vi "LAB3.vi"() -> ()   [LabVIEW 2015]
panel:
  in  "CH2":bool
  in  "CH1":bool
  in  "Enable CH":bool
  out "chaîne résultante 3":string
  out "chaîne résultante 2":string
  out "chaîne en sortie":string
  out "chaîne résultante":string
  out "sortie d'erreur":errorcluster
  in  "Frequency":dbl
  in  "Unit":u16(ring) items=["VPP", "VRMS", "DBM"]
  in  "DC Offset":dbl
  in  "Stop":bool
  in  "Amplitude":dbl
  in  "Waveform":u16(ring) items=["DC", "Sine", "Square", "Ramp", "Pulse", "Noise", "Arb"]
  in  "Configurer":bool
  in  "Nom de ressource VISA":refnum<visa-resource-name>
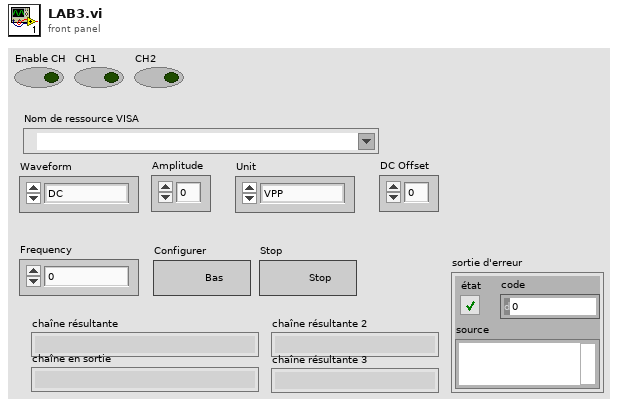
[diagram p1: front panel]
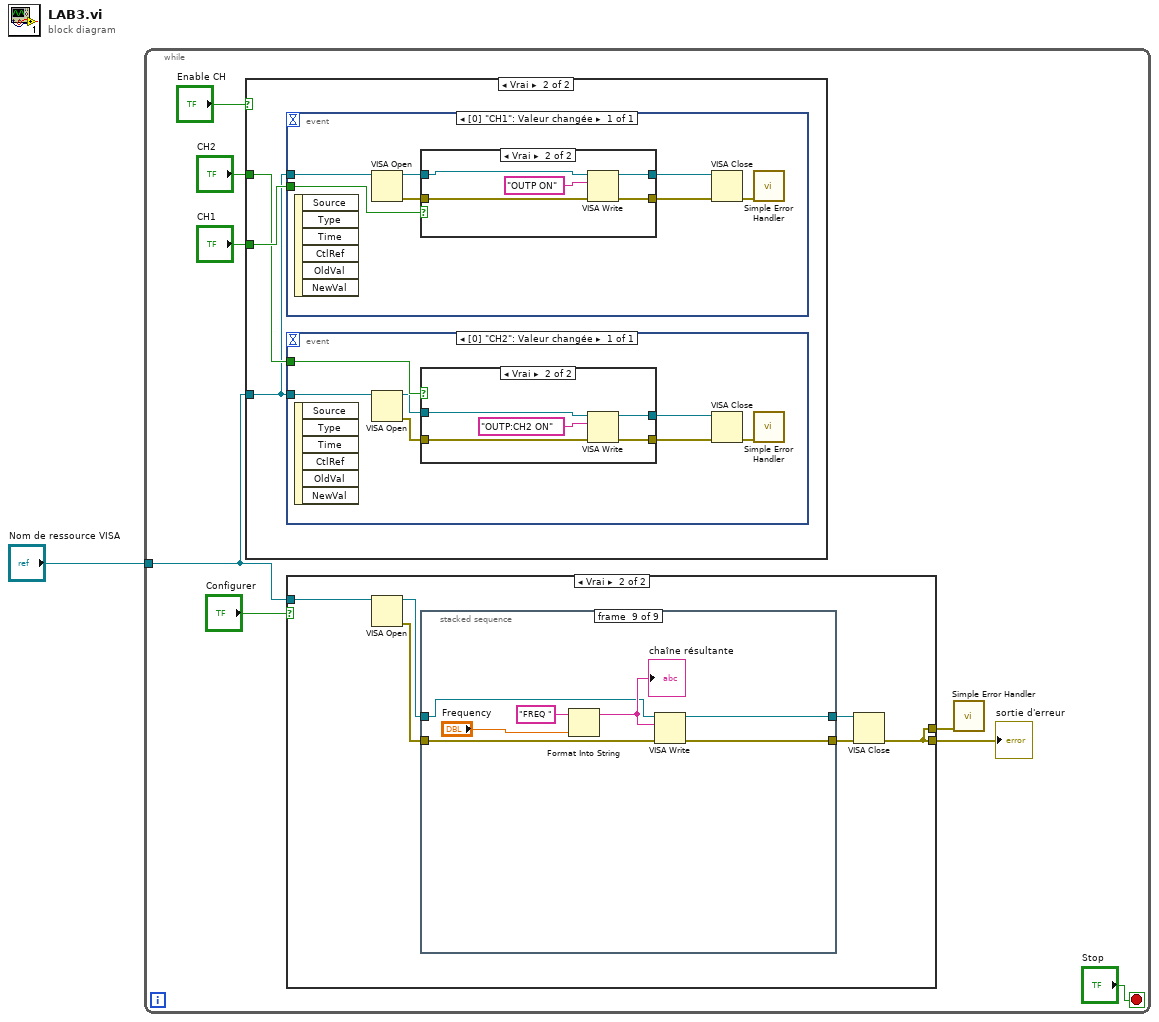
[diagram p0: block diagram]
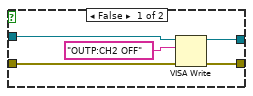
[diagram p3: hidden frame]
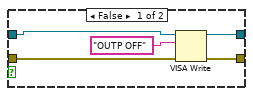
[diagram p4: hidden frame]
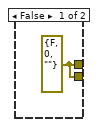
[diagram p5: hidden frame]
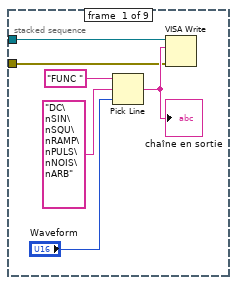
[diagram p6: hidden frame]
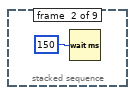
[diagram p7: hidden frame]
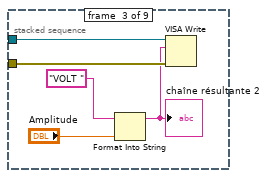
[diagram p8: hidden frame]
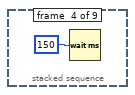
[diagram p9: hidden frame]
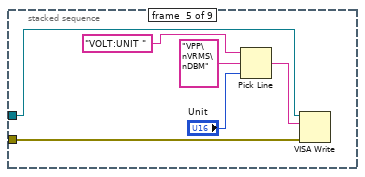
[diagram p10: hidden frame]
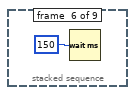
[diagram p11: hidden frame]
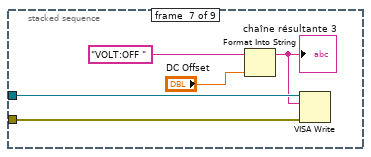
[diagram p12: hidden frame]
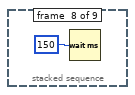
[diagram p13: hidden frame]
diagram:
  n1 = while {
    tunnel: "Nom de ressource VISA" -> [w3]
    stop <- "Stop" stop-if-true
    n2 = case shown="Vrai" "Enable CH" {
      tunnel: "CH1" -> [_ w12]
      tunnel: w3 -> [_ w10]
      tunnel: "CH2" -> [_ w11]
      frame False {
      }
      frame True {
        n3 = event shown="[0] \"CH1\": Valeur changée" {
          selector: _ -> [_]
          dyn-events: _ -> [_]
          timeout: _ -> [_]
          tunnel: w12 -> [w36]
          tunnel: w10 -> [w35]
          event "CH1": Value Change {
            n4 = event-data() -> ()  [unwired: 1 in, 6 out]
            n5 = VISA Open(VISA resource name=w35) -> (VISA resource name=w34:refnum<visa-resource-name>, error out=w33:errorcluster)  [unwired: 4 in]
            n6 = case shown="Vrai" w36 {
              tunnel: w34 -> [w41 w46]
              tunnel: w33 -> [w40 w45]
              tunnel: [w39 w44] -> w32
              tunnel: [w38 w43] -> w31
              frame False {
                n7 = VISA Write(VISA resource name=w41, write buffer="OUTP OFF" ("buffer d'écriture"), error in (no error)=w40) -> (VISA resource name out=w39:refnum<visa-resource-name>, error out=w38:errorcluster)  [unwired: 1 out]
              }
              frame True {
                n8 = VISA Write(VISA resource name=w46, write buffer="OUTP ON" ("buffer d'écriture"), error in (no error)=w45) -> (VISA resource name out=w44:refnum<visa-resource-name>, error out=w43:errorcluster)  [unwired: 1 out]
              }
            }
            n9 = VISA Close(VISA resource name=w32, error in (no error)=w31) -> (error out=w30:errorcluster)
            n10 = call <vilib>:"Simple Error Handler.vi"("error in (no error)"=w30) -> ()  [unwired: 4 in, 5 out]
          }
        }
        n11 = event shown="[0] \"CH2\": Valeur changée" {
          selector: _ -> [_]
          dyn-events: _ -> [_]
          timeout: _ -> [_]
          tunnel: w11 -> [w19]
          tunnel: w10 -> [w18]
          event "CH2": Value Change {
            n12 = event-data() -> ()  [unwired: 1 in, 6 out]
            n13 = VISA Open(VISA resource name=w18) -> (VISA resource name=w17:refnum<visa-resource-name>, error out=w16:errorcluster)  [unwired: 4 in]
            n14 = case shown="Vrai" w19 {
              tunnel: w17 -> [w24 w29]
              tunnel: w16 -> [w23 w28]
              tunnel: [w22 w27] -> w15
              tunnel: [w21 w26] -> w14
              frame False {
                n15 = VISA Write(VISA resource name=w24, write buffer="OUTP:CH2 OFF" ("buffer d'écriture"), error in (no error)=w23) -> (VISA resource name out=w22:refnum<visa-resource-name>, error out=w21:errorcluster)  [unwired: 1 out]
              }
              frame True {
                n16 = VISA Write(VISA resource name=w29, write buffer="OUTP:CH2 ON" ("buffer d'écriture"), error in (no error)=w28) -> (VISA resource name out=w27:refnum<visa-resource-name>, error out=w26:errorcluster)  [unwired: 1 out]
              }
            }
            n17 = VISA Close(VISA resource name=w15, error in (no error)=w14) -> (error out=w13:errorcluster)
            n18 = call <vilib>:"Simple Error Handler.vi"("error in (no error)"=w13) -> ()  [unwired: 4 in, 5 out]
          }
        }
      }
    }
    n19 = case shown="Vrai" "Configurer" {
      tunnel: w3 -> [_ w53]
      tunnel: [w47 w48] -> w9
      tunnel: [w47 w48] -> w6
      frame False {
        w47 = errorcluster {"status"=FALSE, "code"=0, "source"=""} ("error out")
      }
      frame True {
        n20 = VISA Open(VISA resource name=w53) -> (VISA resource name=w52:refnum<visa-resource-name>, error out=w51:errorcluster)  [unwired: 4 in]
        n21 = stacked-sequence {
          tunnel: w52 -> [w56 _ w65 _ w71 _ w78 _ w83]
          tunnel: w51 -> [w54 _ w64 _ w72 _ w77 _ w82]
          tunnel: [_ _ _ _ _ _ _ _ w80] -> w50
          tunnel: [_ _ _ _ _ _ _ _ w81] -> w49
          frame #0 {
            n22 = Pick Line(string ("")="FUNC " ("chaîne (\"\")"), multi-line string="DC\nSIN\nSQU\nRAMP\nPULS\nNOIS\nARB" ("chaîne multiligne"), line index="Waveform") -> (output string=w55:string)
            "chaîne en sortie" <- w55
            n23 = VISA Write(VISA resource name=w56, write buffer=w55, error in (no error)=w54) -> ()  [unwired: 3 out]
          }
          frame #1 {
            n24 = Wait (ms)(milliseconds to wait=u32 150 ("attente (ms)")) -> ()  [unwired: 1 out]
          }
          frame #2 {
            n25 = Format Into String(initial string="VOLT " ("chaîne"), "Amplitude") -> (resulting string=w61:string)  [unwired: 2 in, 1 out]
            "chaîne résultante 2" <- w61
            n26 = VISA Write(VISA resource name=w65, write buffer=w61, error in (no error)=w64) -> ()  [unwired: 3 out]
          }
          frame #3 {
            n27 = Wait (ms)(milliseconds to wait=u32 150 ("attente (ms)")) -> ()  [unwired: 1 out]
          }
          frame #4 {
            n28 = Pick Line(string ("")="VOLT:UNIT " ("chaîne (\"\")"), multi-line string="VPP\nVRMS\nDBM" ("chaîne multiligne"), line index="Unit") -> (output string=w70:string)
            n29 = VISA Write(VISA resource name=w71, write buffer=w70, error in (no error)=w72) -> ()  [unwired: 3 out]
          }
          frame #5 {
            n30 = Wait (ms)(milliseconds to wait=u32 150 ("attente (ms)")) -> ()  [unwired: 1 out]
          }
          frame #6 {
            n31 = Format Into String(initial string="VOLT:OFF " ("chaîne"), "DC Offset") -> (resulting string=w74:string)  [unwired: 2 in, 1 out]
            "chaîne résultante 3" <- w74
            n32 = VISA Write(VISA resource name=w78, write buffer=w74, error in (no error)=w77) -> ()  [unwired: 3 out]
          }
          frame #7 {
            n33 = Wait (ms)(milliseconds to wait=u32 150 ("attente (ms)")) -> ()  [unwired: 1 out]
          }
          frame #8 {
            n34 = Format Into String(initial string="FREQ " ("chaîne initiale"), "Frequency") -> (resulting string=w84:string)  [unwired: 2 in, 1 out]
            "chaîne résultante" <- w84
            n35 = VISA Write(VISA resource name=w83, write buffer=w84, error in (no error)=w82) -> (VISA resource name out=w80:refnum<visa-resource-name>, error out=w81:errorcluster)  [unwired: 1 out]
          }
        }
        n36 = VISA Close(VISA resource name=w50, error in (no error)=w49) -> (error out=w48:errorcluster)
      }
    }
    "sortie d'erreur" <- w6
    n37 = call <vilib>:"Simple Error Handler.vi"("error in (no error)"=w9) -> ()  [unwired: 4 in, 5 out]
  }
